vi "Loop_Auto.vi"() -> ()   [LabVIEW 2017, in "Rotation_Overloard.lvlib"]
uses:
  Rotation_Overloard.lvlib
  _SHARE ALL/Global Share All/Global_STOP.vi
  ENUM_Auto_Action.ctl
  ENUM_Auto_State.ctl
  Arm/ENUM_SM_Rotate_Positions.ctl
  Arm/Arm.lvlib
  Arm/CLUSTER_CMD_SM_Lift_Rotate.ctl
  Claw Rotation/ENUM_SM_Rotate_Positions.ctl
  Claw Rotation/Claw_Rotation.lvlib
  Claw Rotation/CLUSTER_CMD_SM_Lift_Rotate.ctl
  Lift/ENUM_SM_Rotate_Positions.ctl
  Lift/Lift.lvlib
  Lift/CLUSTER_CMD_SM_Lift_Rotate.ctl
  Arm/Global_CMD.vi
  Claw Rotation/Global_CMD.vi
  Lift/Global_CMD.vi
  ENUM_Rotation_Positon.ctl
  CLUSTER_Rotation_CMD.ctl
panel:
  out "Input DBL Data":dbl
  out "Output Bool Data":bool
  out "Output DBL Data":dbl
  out "OutputI INT Data":i32
  out "Cycle Time (S)":dbl format="%.3g"
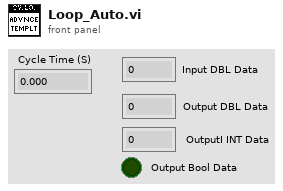
[diagram p1: front panel]
types:
  T1 = typedef "Rotation_Overloard.lvlib/CLUSTER_Rotation_CMD.ctl" = cluster{"Rotation Positon":T2, "Enable Lift":bool}
  T2 = typedef "Rotation_Overloard.lvlib/ENUM_Rotation_Positon.ctl" = enum16{"Starting", "Pickup", "Exchange", "Switch", "Scale", "Climb"}
  T3 = typedef "Lift.lvlib/CLUSTER_CMD_SM_Lift_Rotate.ctl" = cluster{"Enable System":bool, "Rotate Position":T4, "Manual Velocity":dbl, "Manual Mode":bool}
  T4 = typedef "Lift.lvlib/ENUM_SM_Rotate_Positions.ctl" = enum16{"Starting: 0"}
  T5 = typedef "Claw_Rotation.lvlib/CLUSTER_CMD_SM_Lift_Rotate.ctl" = cluster{"Enable System":bool, "Rotate Position":T6, "Manual Velocity":dbl, "Manual Mode":bool}
  T6 = typedef "Claw_Rotation.lvlib/ENUM_SM_Rotate_Positions.ctl" = enum16{"Starting: 0"}
  T7 = typedef "Arm.lvlib/CLUSTER_CMD_SM_Lift_Rotate.ctl" = cluster{"Enable System":bool, "Rotate Position":T8, "Manual Velocity":dbl, "Manual Mode":bool}
  T8 = typedef "Arm.lvlib/ENUM_SM_Rotate_Positions.ctl" = enum16{"Starting: 0"}
  T9 = typedef "Rotation_Overloard.lvlib/ENUM_Auto_State.ctl" = enum16{"Startup", "Idle", "Auto Step 1", "Auto Step 2", "Shutdown"}
  T10 = typedef "Rotation_Overloard.lvlib/ENUM_Auto_Action.ctl" = enum16{"No Action", "Reset Time", "Reset All", "Action A", "Action B"}
  T11 = cluster{"State":T9, "Previous State":T9, "Current Time":timestamp, "Previous Time":timestamp, "Start Time":timestamp, "Target Time (ms)":u32, "Cycle Time(S)":dbl, "Arm CMD":T7, "Claw Rotation CMD":T5, "Lift CMD":T3}
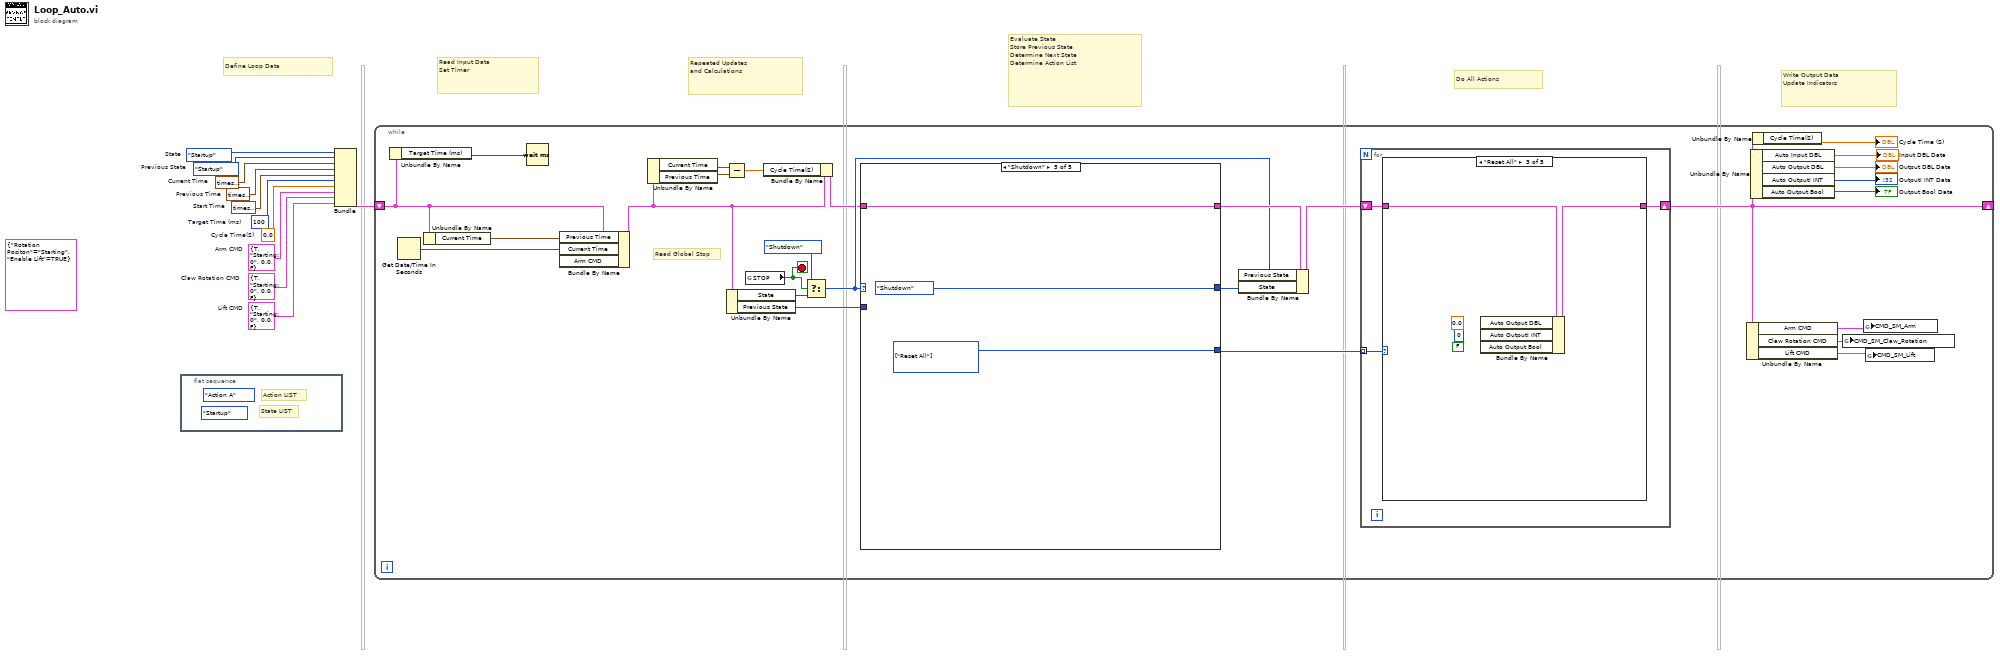
[diagram p0: block diagram]
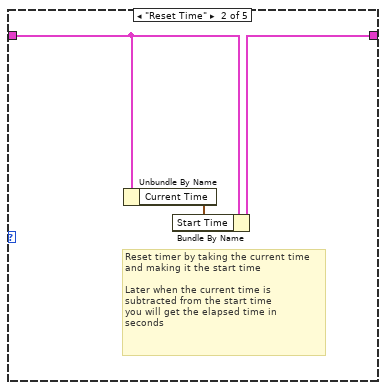
[diagram p3: hidden frame]
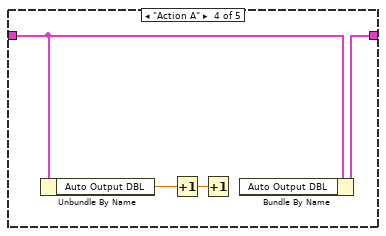
[diagram p4: hidden frame]
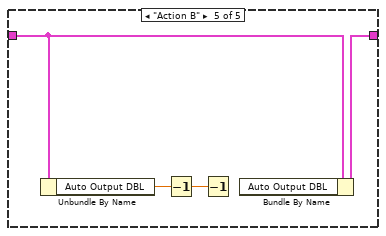
[diagram p5: hidden frame]
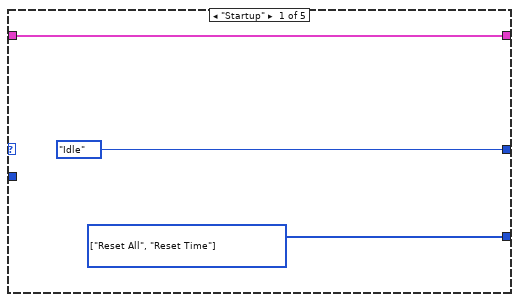
[diagram p6: hidden frame]
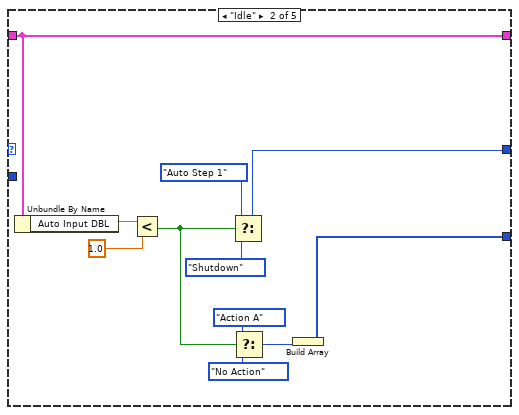
[diagram p7: hidden frame]
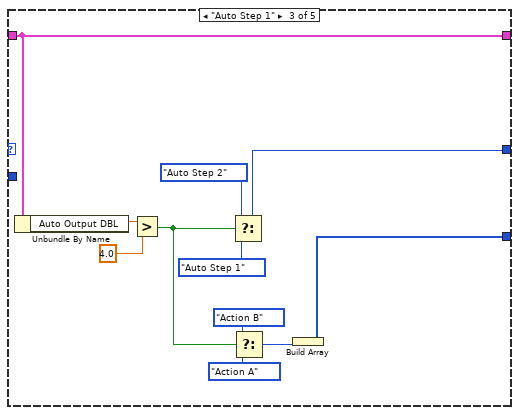
[diagram p8: hidden frame]
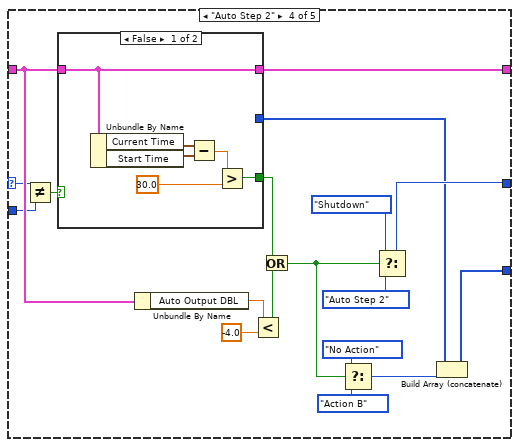
[diagram p9: hidden frame]
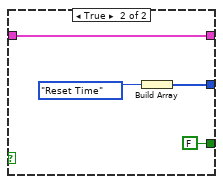
[diagram p10: hidden frame]
diagram:
  (unwired) T1 {"Rotation Positon"=enum."Starting", "Enable Lift"=TRUE}
  w1 = T3 {"Enable System"=TRUE, "Rotate Position"=enum."Starting: 0", "Manual Velocity"=0.0, "Manual Mode"=FALSE}  # Lift CMD
  w2 = T5 {"Enable System"=TRUE, "Rotate Position"=enum."Starting: 0", "Manual Velocity"=0.0, "Manual Mode"=FALSE}  # Claw Rotation CMD
  w3 = T7 {"Enable System"=TRUE, "Rotate Position"=enum."Starting: 0", "Manual Velocity"=0.0, "Manual Mode"=FALSE}  # Arm CMD
  w4 = 0.0  # Cycle Time(S)
  w5 = ENUM_Auto_State."Startup"  # Previous State
  w6 = timestamp(0 s since 1904-01-01)  # Previous Time
  w7 = u32 100  # Target Time (ms)
  w8 = timestamp(0 s since 1904-01-01)  # Start Time
  w9 = timestamp(0 s since 1904-01-01)  # Current Time
  w10 = ENUM_Auto_State."Startup"  # State
  # "Define Loop Data"
  # "Repeated Updates\nand Calculations"
  # "Read Input Data\nSet Timer"
  # "Evaluate State\nStore Previous State\nDetermine Next State\nDetermine Action List"
  # "Do All Actions"
  # "Write Output Data\nUpdate Indicators"
  n1 = flat-sequence {
    frame #0 {
      (unwired) ENUM_Auto_State."Startup" ("State")
      (unwired) ENUM_Auto_Action."Action A" ("Action")
      # "State LIST"
      # "Action LIST"
    }
  }
  n2 = Bundle("State"=w10, "Previous State"=w5, "Current Time"=w9, "Previous Time"=w6, "Start Time"=w8, "Target Time (ms)"=w7, "Cycle Time(S)"=w4, "Arm CMD"=w3, "Claw Rotation CMD"=w2, "Lift CMD"=w1) -> (w11:T11)  [unwired: 1 in]
  n3 = while {
    shift-right: [w24] -> _
    shift-left: w11 -> [w30]
    stop <- w12 stop-if-true
    # "Read Global Stop"
    n4 = Unbundle By Name(w30) -> ("Target Time (ms)"=w32:u32)
    n5 = Get Date/Time In Seconds() -> (seconds since 1Jan1904=w38:timestamp)
    n6 = Unbundle By Name(w30) -> ("Current Time"=w31:timestamp)
    n7 = Wait (ms)(milliseconds to wait=w32) -> ()  [unwired: 1 out]
    n8 = Bundle By Name(cluster=w30, "Previous Time"=w31, "Current Time"=w38) -> (w20:T11)  [unwired: 1 in]
    n9 = Unbundle By Name(w20) -> ("Current Time"=w21:timestamp, "Previous Time"=w22:timestamp)
    n10 = Subtract(x=w21, y=w22) -> (x-y=w18:dbl)
    n11 = Unbundle By Name(w20) -> ("State"=w33:T9, "Previous State"=w29:T9)
    n12 = global read "Global_STOP.vi" "STOP"() -> (w12:bool)
    n13 = Bundle By Name(cluster=w20, "Cycle Time(S)"=w18) -> (w19:T11)
    n14 = Select(t=ENUM_Auto_State."Shutdown" ("State"), s=w12, f=w33) -> (s? t:f=w25:T9)
    n15 = case shown="\"Shutdown\"" w25 {
      selector: w25 -> [_ _ _ w84 _]
      tunnel: w19 -> [w58 w69 w80 w86 w111]
      tunnel: [w58 w69 w80 w85 w111] -> w36
      tunnel: [ENUM_Auto_State."Idle" ("State") w68 w79 w98 ENUM_Auto_State."Shutdown" ("State")] -> w35
      tunnel: [w57 w61 w72 w91 w109] -> w17
      tunnel: w29 -> [_ _ _ w83 _]
      frame "Startup" {
        w57 = T10[] [enum."Reset All", enum."Reset Time"] items=["No Action", "Reset Time", "Reset All", "Action A", "Action B"] ("Actions")
      }
      frame "Idle" {
        n16 = Unbundle By Name(w69) -> ("Auto Input DBL"=w60:dbl)
        n17 = Less?(x=w60, y=1.0) -> (x < y?=w63:bool)
        n18 = Select(t=ENUM_Auto_State."Auto Step 1" ("State"), s=w63, f=ENUM_Auto_State."Shutdown" ("State")) -> (s? t:f=w68:T9)
        n19 = Select(t=ENUM_Auto_Action."Action A" ("Action"), s=w63, f=ENUM_Auto_Action."No Action" ("Action")) -> (s? t:f=w62:T10)
        n20 = Build Array(w62) -> (w61:T10[])
      }
      frame "Auto Step 1" {
        n21 = Unbundle By Name(w80) -> ("Auto Output DBL"=w71:dbl)
        n22 = Greater?(x=w71, y=4.0) -> (0:w74:bool)
        n23 = Select(t=ENUM_Auto_State."Auto Step 2" ("State"), s=w74, f=ENUM_Auto_State."Auto Step 1" ("State")) -> (s? t:f=w79:T9)
        n24 = Select(t=ENUM_Auto_Action."Action B" ("Action"), s=w74, f=ENUM_Auto_Action."Action A" ("Action")) -> (s? t:f=w73:T10)
        n25 = Build Array(w73) -> (w72:T10[])
      }
      frame "Auto Step 2" {
        n26 = Not Equal?(x=w84, y=w83) -> (x != y?=w82:bool)
        n27 = case shown="False" w82 {
          tunnel: [w104 FALSE] -> w93
          tunnel: w86 -> [w99 w107]
          tunnel: [w99 w107] -> w85
          tunnel: [_ w105] -> w81
          frame False {
            n28 = Unbundle By Name(w99) -> ("Current Time"=w102:timestamp, "Start Time"=w101:timestamp)
            n29 = Subtract(x=w102, y=w101) -> (x-y=w100:dbl)
            n30 = Greater?(x=w100, y=30.0) -> (0:w104:bool)
          }
          frame True {
            n31 = Build Array(ENUM_Auto_Action."Reset Time" ("Action")) -> (w105:T10[])
          }
        }
        n32 = Unbundle By Name(w86) -> ("Auto Output DBL"=w89:dbl)
        n33 = Less?(x=w89, y=-4.0) -> (x < y?=w87:bool)
        n34 = Or(x=w93, y=w87) -> (x .or. y?=w90:bool)
        n35 = Select(t=ENUM_Auto_Action."No Action" ("Action"), s=w90, f=ENUM_Auto_Action."Action B" ("Action")) -> (s? t:f=w92:T10)
        n36 = Select(t=ENUM_Auto_State."Shutdown" ("State"), s=w90, f=ENUM_Auto_State."Auto Step 2" ("State")) -> (s? t:f=w98:T9)
        n37 = Build Array (concatenate)(w81, w92) -> (w91:T10[])
      }
      frame "Shutdown" {
        w109 = T10[] [enum."Reset All"] items=["No Action", "Reset Time", "Reset All", "Action A", "Action B"] ("Actions")
      }
    }
    n38 = Bundle By Name(cluster=w36, "Previous State"=w25, "State"=w35) -> (w37:T11)
    n39 = for {
      tunnel: w17 -> [w41] mode=indexing
      shift-right: [w40] -> w24
      shift-left: w37 -> [w39]
      n40 = case shown="\"Reset All\"" w41 {
        tunnel: w39 -> [w42 w45 w47 w50 w54]
        tunnel: [w42 w44 w46 w49 w53] -> w40
        frame "No Action" {
        }
        frame "Reset Time" {
          # "Reset timer by taking the current time\nand making it the start time\n\nLater when the current time is \nsubtracted from the start time\nyou will get the elapsed time in \nseconds"
          n41 = Unbundle By Name(w45) -> ("Current Time"=w43:timestamp)
          n42 = Bundle By Name(cluster=w45, "Start Time"=w43) -> (w44:T11)
        }
        frame "Reset All" {
          (unwired) FALSE ("Output Bool")
          (unwired) 0 ("OutputI INT")
          (unwired) 0.0 ("FG Write Value")
          n43 = Bundle By Name(cluster=w47) -> (w46:T11)  [unwired: 3 in]
        }
        frame "Action A" {
          n44 = Unbundle By Name(w50) -> ("Auto Output DBL"=w51:dbl)
          n45 = Increment(x=w51) -> (x+1=w48:dbl)
          n46 = Increment(x=w48) -> ()  [unwired: 1 out]
          n47 = Bundle By Name(cluster=w50) -> (w49:T11)  [unwired: 1 in]
        }
        frame "Action B" {
          n48 = Unbundle By Name(w54) -> ("Auto Output DBL"=w55:dbl)
          n49 = Decrement(x=w55) -> (x-1=w52:dbl)
          n50 = Decrement(x=w52) -> ()  [unwired: 1 out]
          n51 = Bundle By Name(cluster=w54) -> (w53:T11)  [unwired: 1 in]
        }
      }
    }
    n52 = Unbundle By Name(w24) -> ("Arm CMD"=w15:T7, "Claw Rotation CMD"=w14:T5, "Lift CMD"=w13:T3)
    n53 = Unbundle By Name(w24) -> ("Auto Input DBL"=→"Input DBL Data":dbl, "Auto Output DBL"=→"Output DBL Data":dbl, "Auto OutputI INT"=→"OutputI INT Data":i32, "Auto Output Bool"=→"Output Bool Data":bool)
    n54 = Unbundle By Name(w24) -> ("Cycle Time(S)"=→"Cycle Time (S)":dbl)
    n55 = global write "Global_CMD.vi" "CMD_SM_Claw_Rotation"(w14) -> ()
    n56 = global write "Global_CMD.vi" "CMD_SM_Arm"(w15) -> ()
    n57 = global write "Global_CMD.vi" "CMD_SM_Lift"(w13) -> ()
  }
